vi "AMZ_S3_HMAC-SHA-1 with Base64 encode.vi"(1 "Message":string, 2 "Key":string) -> (0 "Digest (Base64 encoded)":string)   [LabVIEW 2015, in "LV Interface for Amazon S3.lvlib"]
doc: "Signs the Message with Key using HMAC SHA-1 algorithm.\nDigest will be Base64 encoded, because Amazon needs it in that form."
uses:
  LV Interface for Amazon S3.lvlib
  SHA-1/SHA-1.vi
  SHA-1/SHA-1 Core.vi
  SHA-1/SHA-1 Digest.vi
  SHA-1/SHA-1 Pad.vi
  <vilib>/Utility/SMTP/NI_SMTPEmail.lvlib
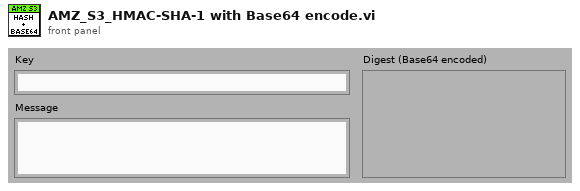
[diagram p1: front panel]
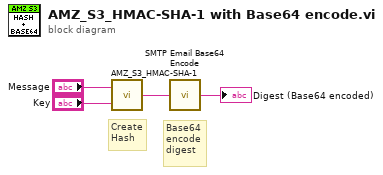
[diagram p0: block diagram]
diagram:
  # "Base64\nencode\ndigest"
  # "Create\nHash"
  n1 = call "AMZ_S3_HMAC-SHA-1.vi"("Key"="Key", "Message"="Message") -> ("Digest"=w4:string)
  n2 = call <vilib>:"SMTP Email Base64 Encode.vi"("Normal String"=w4) -> ("Base64 String"=→"Digest (Base64 encoded)":string)  [unwired: 1 in]
